vi "Close.vi"(8 "Error In":errorcluster, 11 "UDP Ref.":refnum<class "UDP.lvclass">) -> (0 "Error Out":errorcluster)   [LabVIEW 2020, in "RemoteVariables.lvlib" / "UDP.lvclass"]
uses:
  UDP.lvclass
  UDP.lvclass/UDP.ctl
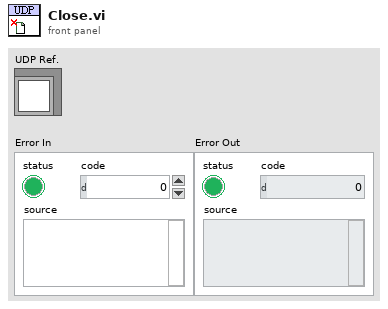
[diagram p1: front panel]
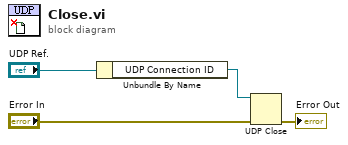
[diagram p0: block diagram]
diagram:
  n1 = Unbundle By Name("UDP Ref.") -> ("UDP Connection ID"=w3:refnum<k16>)
  n2 = UDP Close(connection ID=w3, 8:"Error In") -> (error out=→"Error Out":errorcluster)  [unwired: 1 out]
